vi "Generic_CS.vi"() -> ()   [LabVIEW 2018]
panel:
  out "Graph":u16[](graph)
  in  "stop":bool
  # "Connect proper signal to channel A before starting acquisition\n(e.g. 1Vpp 1kHz sine wave)"
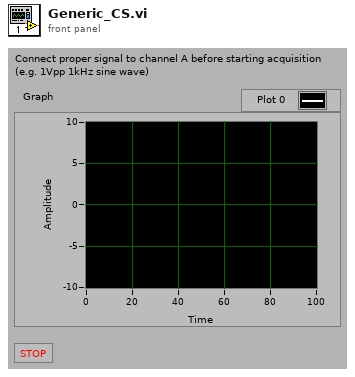
[diagram p1: front panel]
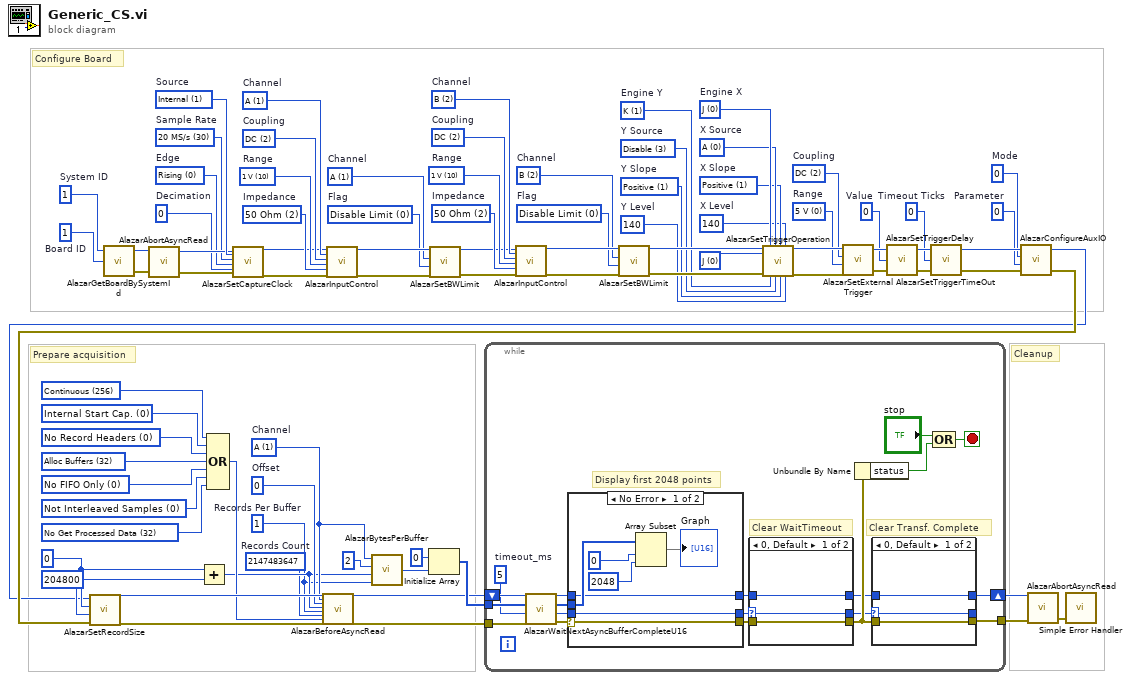
[diagram p0: block diagram]
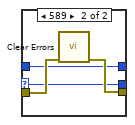
[diagram p2: hidden frame]
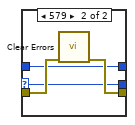
[diagram p3: hidden frame]
diagram:
  w5 = u32 0 items=["No Record Headers"=0, "Enable Record Headers"=8]
  w2 = u32 2147483647  # Records Count
  w1 = u32 1  # Records Per Buffer
  w19 = u32 0  # Offset
  w18 = u32 1 items=["A"=1, "B"=2, "A + B"=3, "C"=4, "A + C"=5, "A + B"=6, "D"=8, "A + D"=9, "B + D"=10, "C + D"=12, "A + B + C + D"=15]  # Channel
  w24 = u32 204800 ("Post-trigger Samples")
  w23 = u32 0 ("Pre-trigger Samples")
  w28 = u32 32 items=["No Get Processed Data"=32, "Get Processed Data"=8192]
  w27 = u32 0 items=["Not Interleaved Samples"=0, "Interleave Samples"=4096]
  w25 = u32 0 items=["No FIFO Only"=0, "FIFO Only"=2048]
  w26 = u32 32 items=["Alloc Buffers"=32]
  w4 = u32 0 items=["Internal Start Cap.", "External Start Cap."]
  w3 = u32 256 items=["Traditional"=0, "NPT"=512, "Continuous"=256, "Triggered Streaming"=1024]
  w58 = u32 0 items=["Disable Limit", "Enable Limit"]  # Flag
  w57 = u32 2 items=["A"=1, "B"=2, "C"=4, "D"=8]  # Channel
  w61 = u32 2 items=["1 MOhm"=1, "50 Ohm"=2]  # Impedance
  w55 = u32 10 items=["20 mV"=1, "40 mV"=2, "50 mV"=3, "80 mV"=4, "100 mV"=5, "200 mV"=6, "400 mV"=7, "500 mV"=8, "800 mV"=9, "1 V"=10, "1.25 V"=33, "2 V"=11, "4 V"=12, "5 V"=13, "8 V"=14, "10 V"=15, "20 V"=16]  # Range
  w62 = u32 2 items=["AC"=1, "DC"=2]  # Coupling
  w63 = u8 2 items=["A"=1, "B"=2, "C"=4, "D"=8]  # Channel
  w31 = u32 0  # Parameter
  w30 = u32 0  # Mode
  w29 = u32 0  # Timeout Ticks
  w36 = u32 0  # Value
  w40 = u32 0 items=["5 V", "1 V", "TTL"]  # Range
  w39 = u32 2 items=["AC"=1, "DC"=2]  # Coupling
  w43 = u32 140  # Y Level
  w44 = u32 1 items=["Positive"=1, "Negative"=2]  # Y Slope
  w45 = u32 3 items=["A", "B", "External", "Disable", "C", "D"]  # Y Source
  w47 = u32 140  # X Level
  w48 = u32 1 items=["Positive"=1, "Negative"=2]  # X Slope
  w49 = u32 0 items=["A", "B", "External", "Disable", "C", "D"]  # X Source
  w46 = u32 1 items=["J", "K"]  # Engine Y
  w50 = u32 0 items=["J", "K"]  # Engine X
  w51 = u32 0 items=["J", "K", "J OR K", "J AND K", "J XOR K", "J AND NOT K", "NOT J AND K"] ("Op.")
  w65 = u32 0 items=["Disable Limit", "Enable Limit"]  # Flag
  w64 = u32 1 items=["A"=1, "B"=2, "C"=4, "D"=8]  # Channel
  w70 = u32 2 items=["1 MOhm"=1, "50 Ohm"=2]  # Impedance
  w71 = u32 10 items=["20 mV"=1, "40 mV"=2, "50 mV"=3, "80 mV"=4, "100 mV"=5, "200 mV"=6, "400 mV"=7, "500 mV"=8, "800 mV"=9, "1 V"=10, "1.25 V"=33, "2 V"=11, "4 V"=12, "5 V"=13, "8 V"=14, "10 V"=15, "20 V"=16]  # Range
  w72 = u32 2 items=["AC"=1, "DC"=2]  # Coupling
  w73 = u8 1 items=["A"=1, "B"=2, "C"=4, "D"=8]  # Channel
  w75 = u32 0  # Decimation
  w76 = u32 0 items=["Rising", "Falling"]  # Edge
  w77 = u32 30 items=["1 kS/s"=1, "2 kS/s"=2, "5 kS/s"=4, "10 kS/s"=8, "20 kS/s"=10, "50 kS/s"=12, "100 kS/s"=14, "200 kS/s"=16, "500 kS/s"=18, "1 MS/s"=20, "2 MS/s"=24, "5 MS/s"=26, "10 MS/s"=28, "20 MS/s"=30, "25 MS/s"=33, "50 MS/s"=34, "100 MS/s"=36, "125 MS/s"=37, "160 MS/s"=38, "180 MS/s"=39, "250 MS/s"=43, "500 MS/s"=48, "800 MS/s"=50, "1000 MS/s"=53, "1200 MS/s"=55, "1500 MS/s"=58, "1800 MS/s"=61, "USER_DEF"=0]  # Sample Rate
  w79 = u32 1 items=["Internal"=1, "Fast External"=2, "Medium External"=3, "Slow External"=4, "External AC"=5, "External DC"=6, "External 10MHz"=7]  # Source
  w83 = u32 1  # Board ID
  w82 = u32 1  # System ID
  # "Cleanup"
  # "Prepare acquisition"
  # "Configure Board"
  n1 = call "AlazarGetBoardBySystemId.vi"("Board ID"=w83, "System ID"=w82) -> ("error out"=w80:errorcluster, "Handle"=w81:u64)  [unwired: 1 in, 1 out]
  n2 = call "AlazarAbortAsyncRead.vi"("Handle"=w81, "error in (no error)"=w80) -> ("Handle"=w78:u64, "error out"=w74:errorcluster)  [unwired: 1 out]
  n3 = Add(x=w23, y=w24) -> (x+y=w6:u32)
  n4 = Compound Arithmetic op=OR(w3, w4, w5, w26, w25, w27, w28) -> (w20:u32)
  n5 = call "AlazarSetCaptureClock.vi"("Handle"=w78, "Source"=w79, "Sample Rate"=w77, "Edge"=w76, "Decimation"=w75, "error in (no error)"=w74) -> ("Handle"=w69:u64, "error out"=w68:errorcluster)  [unwired: 11 in, 1 out]
  n6 = call "AlazarInputControl.vi"("Handle"=w69, "Channel"=w73, "Coupling"=w72, "Range"=w71, "Impedance"=w70, "error in (no error)"=w68) -> ("Handle"=w67:u64, "error out"=w66:errorcluster)  [unwired: 11 in, 1 out]
  n7 = call "AlazarBytesPerBuffer.vi"("Records Per Buffer"=w1, "Samples Per Record"=w6, "Bytes Per Sample"=u32 2, "Channel Mask"=w18) -> ("Bytes Per Buffer"=w16:u32)
  n8 = Initialize Array(u16 0, w16) -> (w14:u16[])
  n9 = call "AlazarSetBWLimit.vi"("error in (no error)"=w66, "Flag"=w65, "Channel"=w64, "Handle"=w67) -> ("error out"=w56:errorcluster, "Handle"=w54:u64)  [unwired: 1 out]
  n10 = call "AlazarInputControl.vi"("Handle"=w54, "Channel"=w63, "Coupling"=w62, "Range"=w55, "Impedance"=w61, "error in (no error)"=w56) -> ("Handle"=w60:u64, "error out"=w59:errorcluster)  [unwired: 11 in, 1 out]
  n11 = call "AlazarSetBWLimit.vi"("error in (no error)"=w59, "Flag"=w58, "Channel"=w57, "Handle"=w60) -> ("error out"=w52:errorcluster, "Handle"=w53:u64)  [unwired: 1 out]
  n12 = call "AlazarSetTriggerOperation.vi"("Handle"=w53, "Trigger Operation"=w51, "error in (no error)"=w52, "Trigger Engine 1"=w50, "Trigger Engine 2"=w46, "Source 1"=w49, "Source 2"=w45, "Slope 1"=w48, "Slope 2"=w44, "Level 1"=w47, "Level 2"=w43) -> ("Handle"=w42:u64, "error out"=w41:errorcluster)  [unwired: 6 in, 1 out]
  n13 = call "AlazarSetExternalTrigger.vi"("error in (no error)"=w41, "Range ID"=w40, "Coupling ID"=w39, "Handle"=w42) -> ("error out"=w37:errorcluster, "Handle"=w38:u64)  [unwired: 1 out]
  n14 = call "AlazarSetTriggerDelay.vi"("error in (no error)"=w37, "Delay"=w36, "Handle"=w38) -> ("error out"=w34:errorcluster, "Handle"=w35:u64)  [unwired: 1 out]
  n15 = call "AlazarSetTriggerTimeOut.vi"("error in (no error)"=w34, "Timeout Ticks"=w29, "Handle"=w35) -> ("error out"=w32:errorcluster, "Handle"=w33:u64)  [unwired: 1 out]
  n16 = call "AlazarConfigureAuxIO.vi"("error in (no error)"=w32, "Parameter"=w31, "Mode"=w30, "Handle"=w33) -> ("error out"=w8:errorcluster, "Handle"=w7:u64)  [unwired: 1 out]
  n17 = call "AlazarSetRecordSize.vi"("error in (no error)"=w8, "Post-trigger Samples"=w24, "Pre-trigger Samples"=w23, "Handle"=w7) -> ("error out"=w21:errorcluster, "Handle"=w22:u64)  [unwired: 1 out]
  n18 = call "AlazarBeforeAsyncRead.vi"("Handle"=w22, "Channel Select"=w18, "Transfer Offset"=w19, "Transfer Length"=w6, "Records Per Buffer"=w1, "Records Per Acquisition"=w2, "Flags"=w20, "error in (no error)"=w21) -> ("Handle"=w13:u64, "error out"=w12:errorcluster)  [unwired: 17 in, 1 out]
  n19 = while {
    tunnel: w14 -> [w102]
    tunnel: w12 -> [w99]
    tunnel: [w87] -> w9
    shift-right: [w88] -> w10
    shift-left: w13 -> [w101]
    stop <- w84 stop-if-true
    w100 = u32 5  # timeout_ms
    # "Clear Transf. Complete"
    # "Clear WaitTimeout"
    # "Display first 2048 points"
    n20 = call "AlazarWaitNextAsyncBufferCompleteU16.vi"("error in (no error)"=w99, "Timeout (ms)"=w100, "Buffer"=w102, "Handle"=w101) -> ("error out"=w98:errorcluster, "Return Code"=w97:u32, "Buffer"=w92:u16[], "Handle"=w94:u64)
    n21 = case shown="No Error" w98 {
      selector: w98 -> [w117 w125]
      tunnel: w97 -> [w119 w126]
      tunnel: [w119 w126] -> w96
      tunnel: [w117 w125] -> w95
      tunnel: [w118 w124] -> w93
      tunnel: w94 -> [w118 w124]
      tunnel: w92 -> [w122 _]
      frame No Error {
        n22 = Array Subset(array=w122, index=0, length=2048) -> (→"Graph":u16[])
      }
      frame Error {
      }
    }
    n23 = case shown="0, Default" w96 {
      selector: w96 -> [w111 w113]
      tunnel: w95 -> [w110 w116]
      tunnel: [w110 w115] -> w91
      tunnel: [w112 w114] -> w90
      tunnel: w93 -> [w112 w114]
      tunnel: [w111 w113] -> w89
      frame 0, Default {
      }
      frame 579 {
        n24 = call <vilib>:"Clear Errors.vi"("error in (no error)"=w116) -> ("error out"=w115:errorcluster)  [unwired: 5 in, 1 out]
      }
    }
    n25 = Unbundle By Name(w91) -> ("status"=w86:bool)
    n26 = case shown="0, Default" w89 {
      selector: w89 -> [w104 w106]
      tunnel: w91 -> [w103 w109]
      tunnel: [w103 w108] -> w87
      tunnel: [w105 w107] -> w88
      tunnel: w90 -> [w105 w107]
      tunnel: [w104 w106] -> _
      frame 0, Default {
      }
      frame 589 {
        n27 = call <vilib>:"Clear Errors.vi"("error in (no error)"=w109) -> ("error out"=w108:errorcluster)  [unwired: 5 in, 1 out]
      }
    }
    n28 = Compound Arithmetic op=OR("stop", w86) -> (w84:bool)
  }
  n29 = call "AlazarAbortAsyncRead.vi"("Handle"=w10, "error in (no error)"=w9) -> ("error out"=w11:errorcluster)  [unwired: 2 out]
  n30 = call <vilib>:"Simple Error Handler.vi"("error in (no error)"=w11) -> ()  [unwired: 4 in, 5 out]
